vi "mak_balaji_loop.vi"() -> ()   [LabVIEW 2014]
doc: "this vi has a clock which has two indicators \n\ngreen- moves(technicaly Bit 1 is swaped to produce an optical illusion that the pointer moves 90 dgree clockwise ) when 0.25 second is counted.\n\nred- moves when 15 second is counted.\n\nif the counted time exceeds 60 second(1 minute) then the program status is changed to OVERFLOW. (user can also intrupt the counting operation and can stop the clock) \n\nCreated by \nBalaji V \nfor the purpose of learning about functions of loops(while & for)\nand it is submitted to the makcontrols india pvt ltd for the purpose of verification"
panel:
  out "Program status":string
  in  "?":bool
  out "seconds":dbl
  out "0 S":bool
  out "45 S":bool
  out "30 S":bool
  out "15 S":bool
  out "H S":bool
  out "Z S":bool
  out "3Q S":bool
  out "Q S":bool
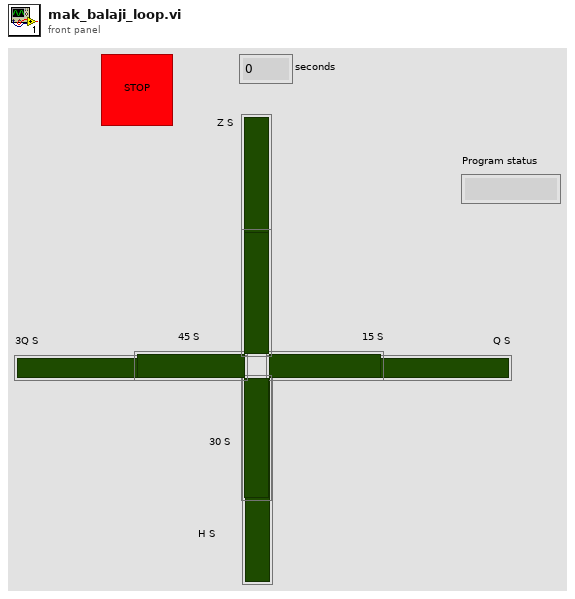
[diagram p1: front panel]
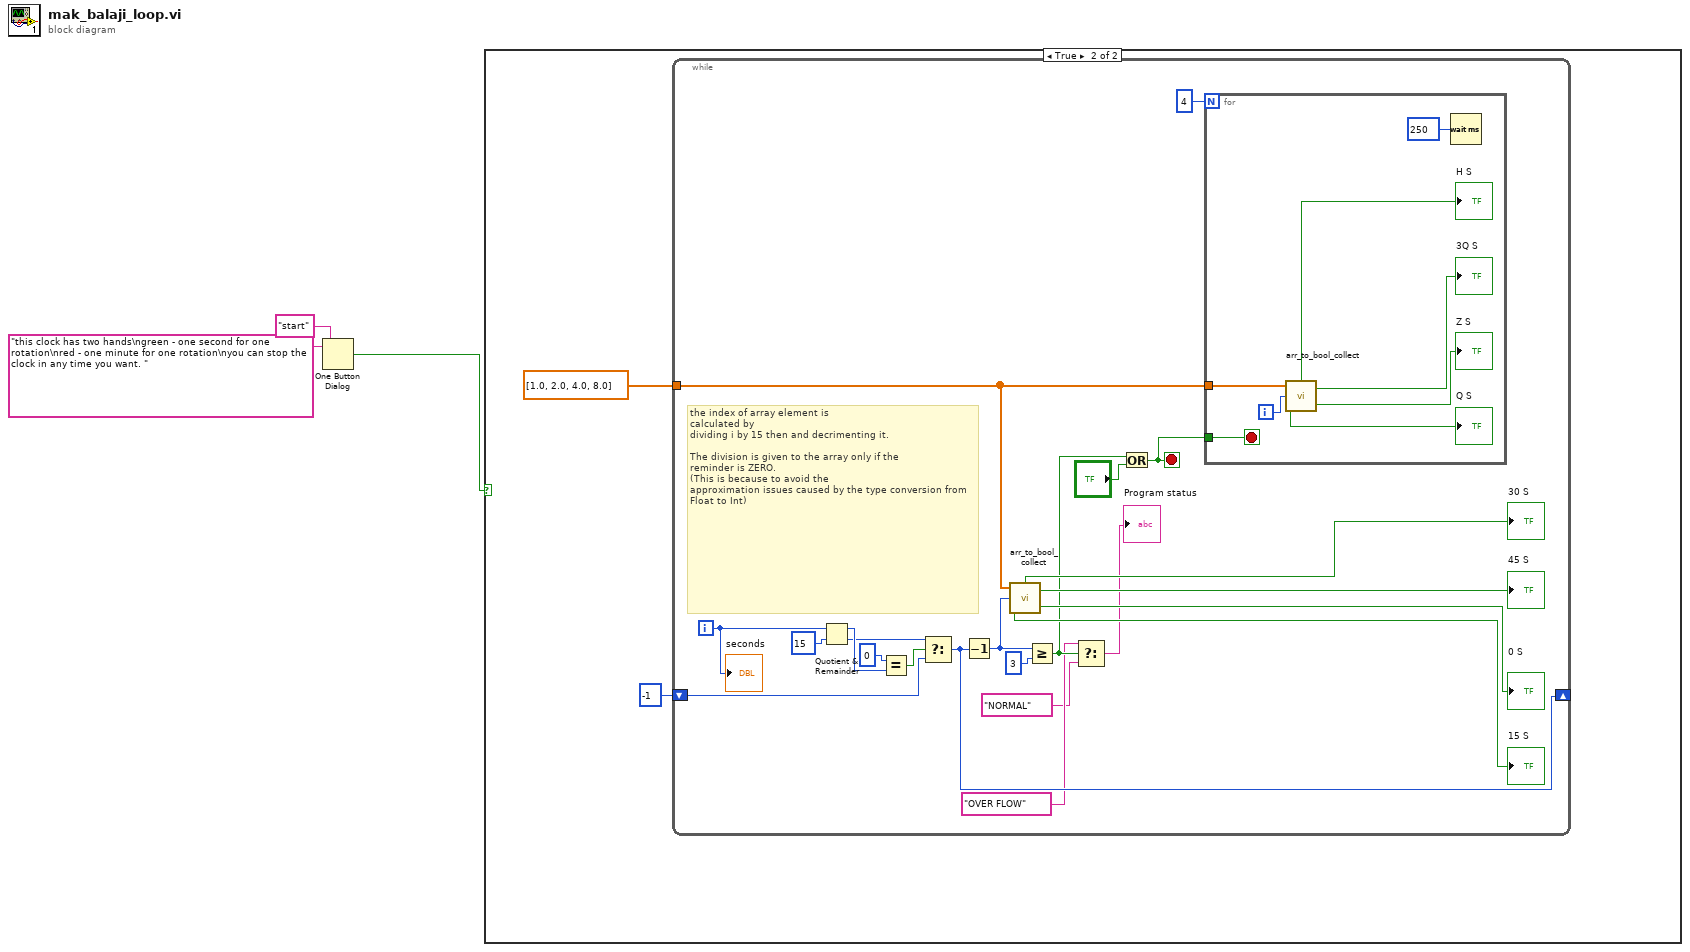
[diagram p0: block diagram]
diagram:
  n1 = One Button Dialog(message="this clock has two hands\ngreen - one second for one rotation\nred - one minute for one rotation\nyou can stop the clock in any time you want. ", button name ("OK")="start") -> (true=w3:bool)
  n2 = case shown="True" w3 {
    frame False {
    }
    frame True {
      n3 = while {
        tunnel: dbl[] [1.0, 2.0, 4.0, 8.0] ("array") -> [w26]
        shift-right: [w14] -> _
        shift-left: -1 -> [w16]
        i -> [w21]
        stop <- w10 stop-if-true
        # "the index of array element is\ncalculated by\ndividing i by 15 then and decrimenting it.\n\nThe division is given to the array only if the\nreminder is ZERO.\n(This is because to avoid the \napproximation issues caused by the type conversion from Float to Int)"
        n4 = Quotient & Remainder(x=w21, y=15) -> (x-y*floor(x/y)=w19:i32, floor(x/y)=w15:i32)
        n5 = Equal?(x=0, y=w19) -> (x = y?=w17:bool)
        n6 = Select(t=w15, s=w17, f=w16) -> (s? t:f=w14:i32)
        n7 = Decrement(x=w14) -> (x-1=w13:i32)
        n8 = call "arr_to_bool_collect.vi"("index"=w13, "array"=w26) -> ("Boolean array[3]"=→"0 S":bool, "Boolean array[2]"=→"45 S":bool, "Boolean array[1]"=→"30 S":bool, "Boolean array[0]"=→"15 S":bool)
        n9 = Greater Or Equal?(x=w13, y=3) -> (x >= y?=w9:bool)
        n10 = Select(t="OVER FLOW", s=w9, f="NORMAL") -> (s? t:f=→"Program status":string)
        n11 = Or(x=w9, y="?") -> (x .or. y?=w10:bool)
        n12 = for {
          N: 4 -> [_]
          tunnel: w26 -> [w34]
          tunnel: w10 -> [w28]
          i -> [w33]
          stop <- w28 stop-if-true
          n13 = call "arr_to_bool_collect.vi"("index"=w33, "array"=w34) -> ("Boolean array[3]"=→"Z S":bool, "Boolean array[2]"=→"3Q S":bool, "Boolean array[1]"=→"H S":bool, "Boolean array[0]"=→"Q S":bool)
          n14 = Wait (ms)(milliseconds to wait=u32 250) -> ()  [unwired: 1 out]
        }
        "seconds" <- w21
      }
    }
  }
